vi "InitActor.vi"(8 "error in (no error)":errorcluster, 10 "InitData":T2, 11 "CameraTestingCI in":refnum<class "CameraTestingENI.lvclass">) -> (0 "error out":errorcluster, 3 "CameraTestingCI out":refnum<class "CameraTestingENI.lvclass">)   [LabVIEW 2020, in "CameraTestingProxy.lvlib" / "CameraTestingENI.lvclass"]
uses:
  CameraTestingENI.lvclass
  CameraTestingENI.lvclass/CameraTestingENI.ctl
  Camera/ICamera/ICamera/ICamera.lvclass
  TypeDef/RequestEventList.ctl
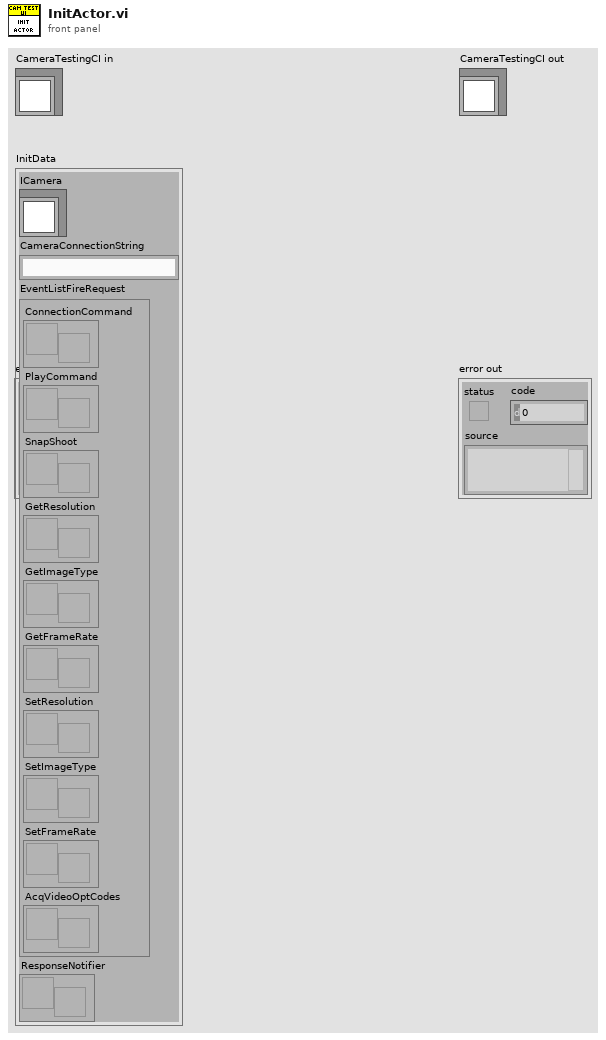
[diagram p1: front panel]
types:
  T1 = typedef "CameraTestingProxy.lvlib/CameraTestingENI.lvclass/RequestEventList.ctl" = cluster{"ConnectCmd":refnum<user-event>, "PlayCmd":refnum<user-event>, "SnapShoot":refnum<user-event>, "GetResolution":refnum<user-event>, "GetImageType":refnum<user-event>, "GetFrameRate":refnum<user-event>, "SetResolution":refnum<user-event>, "SetImageType":refnum<user-event>, "SetFrameRate":refnum<user-event>, "AcqVideoOptCodes":refnum<user-event>}
  T2 = cluster{"ICamera":refnum<class "ICamera.lvclass">, "CamConnStr":string, "EvnListFireRqst":T1, "ResponseNotifier":refnum<notifier>}
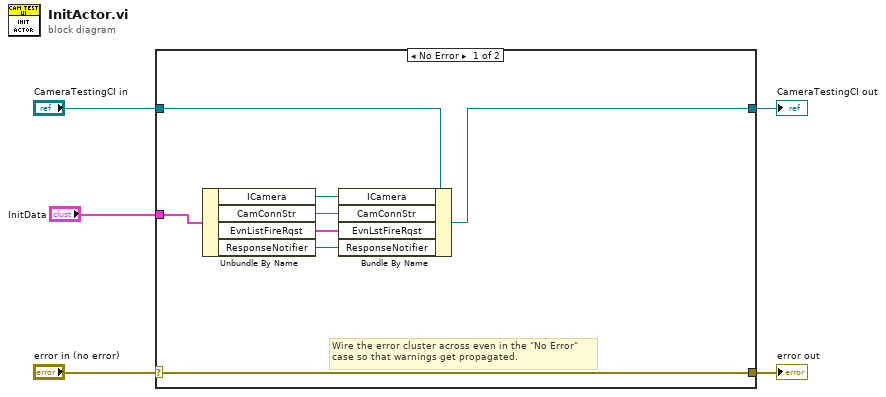
[diagram p0: block diagram]
diagram:
  n1 = case shown="No Error" "error in (no error)" {
    selector: "error in (no error)" -> [w13 w15]
    tunnel: [w13 w15] -> w4
    tunnel: [w11 w14] -> w2
    tunnel: "CameraTestingCI in" -> [w12 w14]
    tunnel: "InitData" -> [w10 _]
    frame No Error {
      # "Wire the error cluster across even in the \"No Error\"\ncase so that warnings get propagated."
      n2 = Unbundle By Name(w10) -> ("ICamera"=w9:refnum<class "ICamera.lvclass">, "CamConnStr"=w8:string, "EvnListFireRqst"=w7:T1, "ResponseNotifier"=w6:refnum<notifier>)
      n3 = Bundle By Name(cluster=w12, "ICamera"=w9, "CamConnStr"=w8, "EvnLstFireRqst"=w7, "ResponseNotifier"=w6) -> (w11:refnum<class "CameraTestingENI.lvclass">)
    }
    frame Error {
    }
  }
  "error out" <- w4
  "CameraTestingCI out" <- w2
